vi "Autonomous Independent.vi"   [LabVIEW 2016]
doc: "This VI is called when autonomous begins, and will automatically be terminated when autonomous ends. You can carry out timed or sensor driven robot movement independently without needing to return to the caller."
uses:
  <vilib>/Rock Robotics/WPI/DriverStation/WPI_DriverStationRobotMode2.ctl
  <vilib>/Rock Robotics/WPI/Utilities/WPI_GetSetVariantRefNum.vi
  <vilib>/Rock Robotics/Network Tables/NT Read String.vi
  <vilib>/Rock Robotics/Network Tables/NT Read Number.vi
  Robot Global Data.vi
  <vilib>/Rock Robotics/Network Tables/NT Write Numeric Array.vi
panel:
  # "Be sure to right-click and choose Data Operations>>Make Current Value default if you want to save the array values with the VI"
types:
  T1 = typedef "WPI_JoystickDevRef.ctl" = cluster{"Device":T2}
  T2 = typedef "WPI_JoystickDeviceEnum.ctl" = enum16{"USB 0", "USB 1", "USB 2", "USB 3", "USB 4", "USB 5"}
  T3 = typedef "WPI_DriverStationRobotMode2.ctl" = enum16{"Autonomous Disabled", "Autonomous Enabled", "Teleop Disabled", "Teleop Enabled", "Disconnected", "Finish", "Test Disabled", "Test Enabled", "Emergency Stopped"}
  T4 = typedef "WPI_RobotDriveDevRef.ctl" = cluster{"DevStatus":errorcluster, "Motors[]":T5[], "Square Inputs":bool, "Max Output":dbl}
  T5 = typedef "WPI_MotorControlDeviceRef.ctl" = cluster{"DeviceStatus":errorcluster, "Type":T6, "PWM":cluster{"PWM Channel":T7, "DeadBand":T8}, "CAN":cluster{"Device Number":u8, "SetOutput VI Ref":variant, "GetOutput VI Ref":variant, "Enable VI Ref":variant, "Disable VI Ref":variant, "Data":variant}, "Invert":bool}
  T6 = typedef "WPI_MotorControlType.ctl" = enum16{"PWM", "CAN"}
  T7 = typedef "FPGA_DIOPWMChannel.ctl" = enum8{"PWM 0", "PWM 1", "PWM 2", "PWM 3", "PWM 4", "PWM 5", "PWM 6", "PWM 7", "PWM 8", "PWM 9", "PWM MXP 0", "PWM MXP 1", "PWM MXP 2", "PWM MXP 3", "PWM MXP 4", "PWM MXP 5", "PWM MXP 6", "PWM MXP 7", "PWM MXP 8", "PWM MXP 9", "Invalid"}
  T8 = typedef "WPI_PWMDeadband.ctl" = cluster{"Name":string, "maxPositivePwm":i32, "minPositivePwm":i32, "centerPwm":i32, "maxNegativePwm":i32, "minNegativePwm":i32, "angularRange":u16}
  T9 = typedef "WPI_ServoDeviceRef.ctl" = cluster{"DeviceStatus":errorcluster, "PWM Channel":T7, "DeadBand":T8}
  T10 = typedef "WPI_CANTalonSRX_GlobalStatus.ctl" = cluster{"Applied Throttle":dbl, "Module Enabled":bool, "CAN Error":errorcluster, "Closed Loop Error":dbl, "Forward Limit Switch Closed":bool, "Reverse Limit Switch Closed":bool, "Sensor Position":dbl, "Sensor Velocity":dbl, "Current":dbl, "Sticky Fault - Over Temp":bool, "Sticky Fault - Under Voltage":bool, "Sticky Fault - Forward Limit":bool, "Sticky Fault - Reverse Limit":bool, "Sticky Fault - Forward Soft Limit":bool, "Sticky Fault - Reverse Soft Limit":bool, "Brake is Enabled":bool, "Encoder Position":dbl, "Encoder Velocity":dbl, "Encoder Index Count":dbl, "Encoder A Pin State":bool, "Encoder B Pin State":bool, "Encoder Index Pin State":bool, "Analog In":dbl, "Analog In Velocity":dbl, "Temperature (C)":dbl, "Battery Voltage":dbl, "Control 5 Is Supported":bool, "Current Profile Slot Select":dbl, "Pos Div 8":bool, "Vel Div 4":bool, "Pulse Width Position":i32, "Pulse Width Velocity":i32, "Pulse Width Rise To Rise (us)":i32, "Pulse Width Rise To Fall (us)":i32, "Mot Prof Active Is Under Run":bool, "Mot Prof Active Has Under Run":bool, "Mot Prof Active Is Last":bool, "Mot Prof Active Velocity Only":bool, "Mot Prof Active Is Valid":bool, "Mot Prof Buffer Is Full":bool, "Mot Prof Active Profile Slot Select":i32, "Mot Prof NextID":i32, "Mot Prof Count":i32, "Mot Prof Active Velocity":dbl, "Mot Prof Active Position":dbl, "Mot Prof Output Enable":i32}
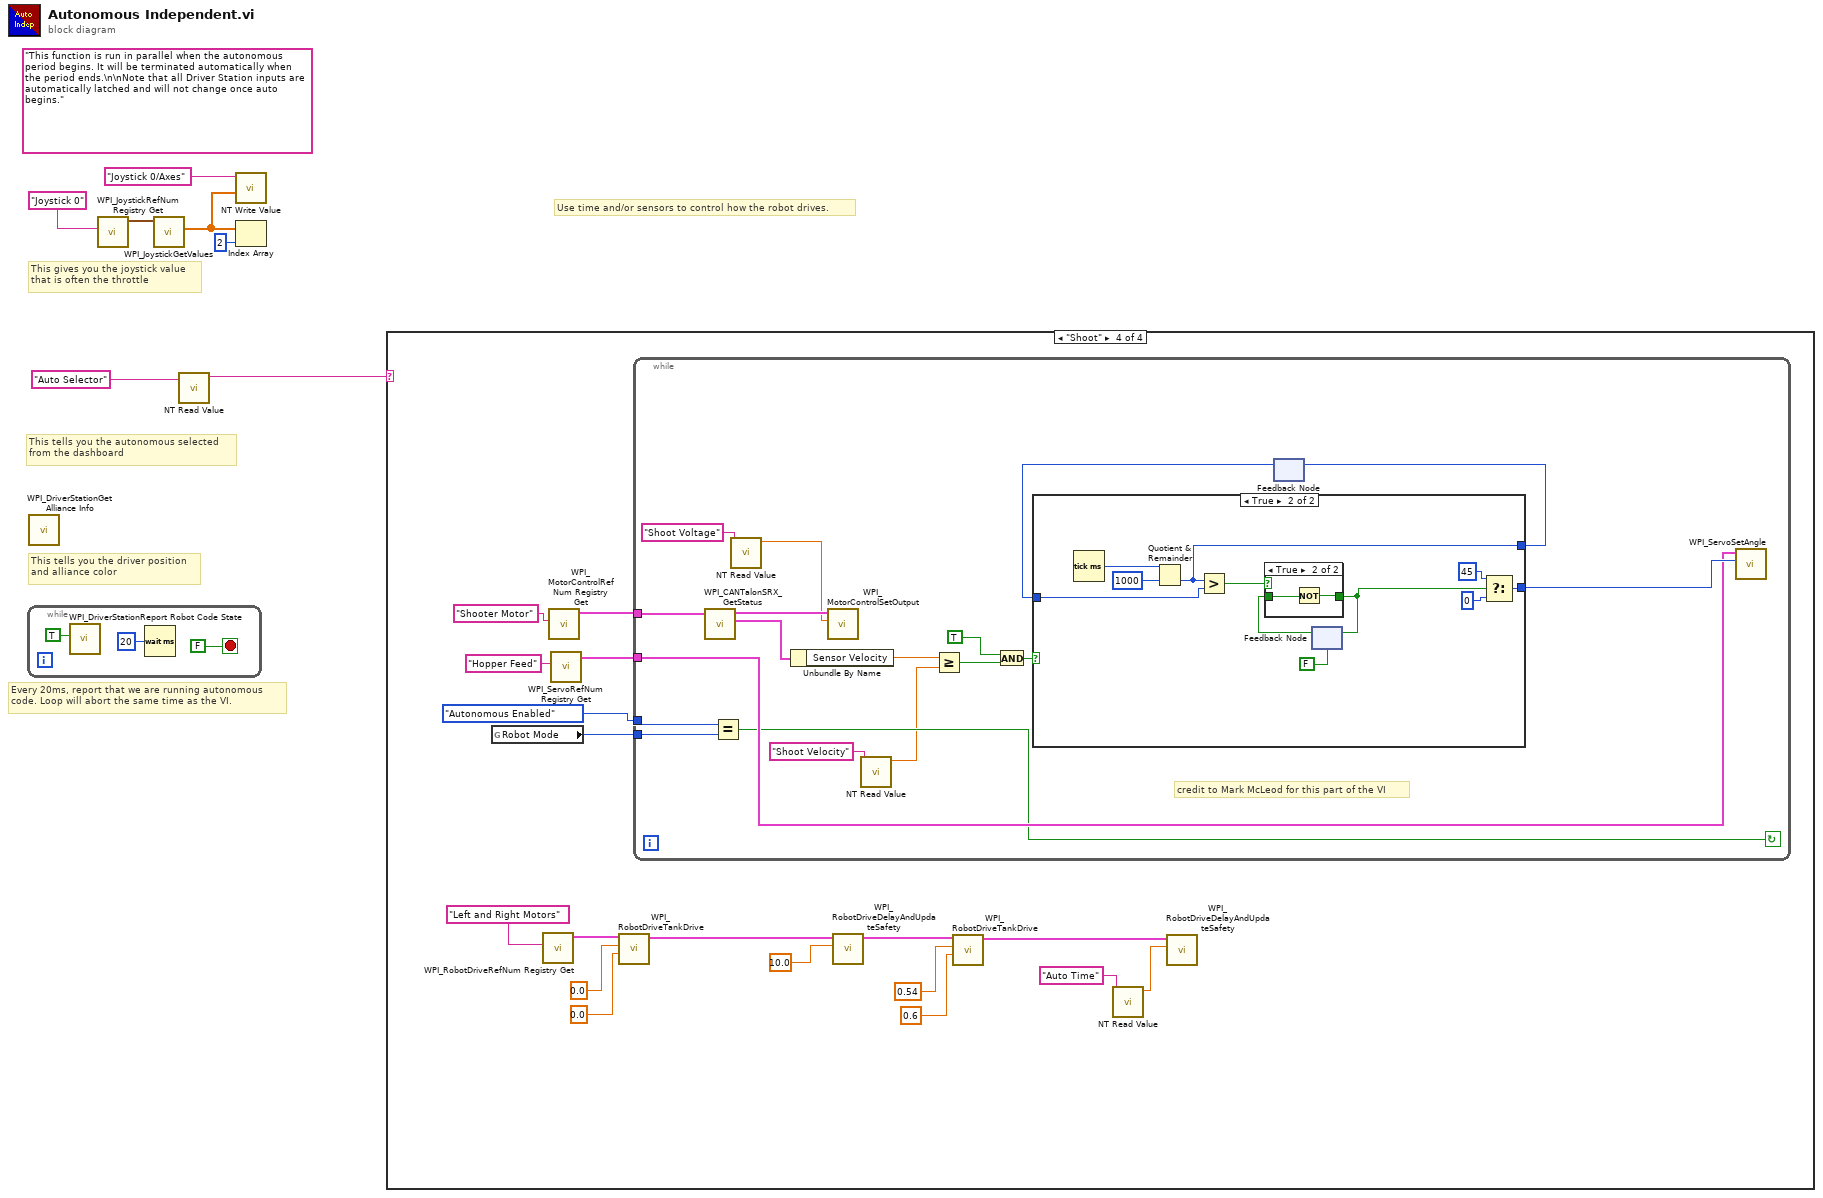
[diagram p0: block diagram]
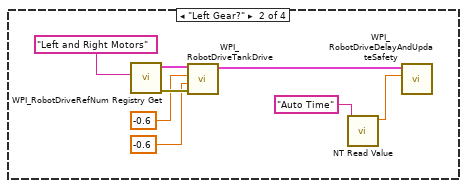
[diagram p3: hidden frame]
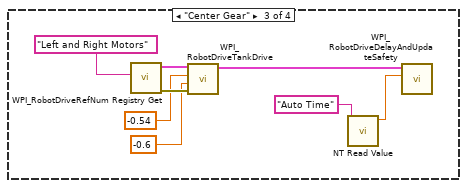
[diagram p4: hidden frame]
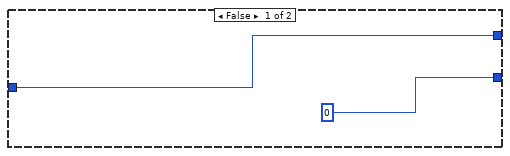
[diagram p5: hidden frame]
diagram:
  (unwired) "This function is run in parallel when the autonomous period begins. It will be terminated automatically when the period ends.\n\nNote that all Driver Station inputs are automatically latched and will not change once auto begins."
  # "This tells you the autonomous selected\nfrom the dashboard"
  # "Every 20ms, report that we are running autonomous\ncode. Loop will abort the same time as the VI."
  # "This gives you the joystick value\nthat is often the throttle"
  # "Use time and/or sensors to control how the robot drives."
  # "This tells you the driver position\nand alliance color"
  n1 = while {
    stop <- FALSE stop-if-true
    n2 = call <vilib>:"WPI_DriverStationReport Robot Code State.vi"("Autonomous"=TRUE) -> ()  [unwired: 10 in, 1 out]
    n3 = Wait (ms)(milliseconds to wait=u32 20) -> ()  [unwired: 1 out]
  }
  n4 = call <vilib>:"WPI_DriverStationGet Alliance Info.vi"() -> ()  [unwired: 12 out]
  n5 = call <vilib>:"WPI_JoystickRefNum Registry Get.vi"("refnum name"="Joystick 0") -> ("JoystickDevRef"=w6:T1)  [unwired: 1 in, 9 out]
  n6 = call <vilib>:"WPI_JoystickGetValues.vi"("JoystickDevRef"=w6) -> ("Axes"=w3:dbl[])  [unwired: 6 in, 4 out]
  n7 = call-poly <vilib>:"NT Read Value.vi"("Name"="Auto Selector") -> ("String"=w1:string)  [unwired: 9 in, 1 out]
  n8 = call-poly <vilib>:"NT Write Value.vi"("Numeric Array"=w3, "Name"="Joystick 0/Axes") -> ()  [unwired: 9 in, 1 out]
  n9 = Index Array(array=w3, index=2) -> ()  [unwired: 1 out]
  n10 = case shown="\"Shoot\"" w1 {
    frame Default {
    }
    frame "Left Gear?" {
      n11 = call <vilib>:"WPI_RobotDriveRefNum Registry Get.vi"("refnum name"="Left and Right Motors") -> ("error out"=w17:errorcluster, "RobotDriveDevRef"=w16:T4)  [unwired: 1 in, 8 out]
      n12 = call <vilib>:"WPI_RobotDriveTankDrive.vi"("error in (no error)"=w17, "Right axis value"=-0.6, "Left axis value"=-0.6, "RobotDriveDevRef"=w16) -> ("RobotDriveDevRef"=w13:T4)  [unwired: 5 in, 2 out]
      n13 = call-poly <vilib>:"NT Read Value.vi"("Name"="Auto Time") -> ("Numeric"=w12:dbl)  [unwired: 9 in, 1 out]
      n14 = call <vilib>:"WPI_RobotDriveDelayAndUpdateSafety.vi"("Delay (s)"=w12, "RobotDriveDevRef"=w13) -> ()  [unwired: 8 in, 2 out]
    }
    frame "Center Gear" {
      n15 = call <vilib>:"WPI_RobotDriveRefNum Registry Get.vi"("refnum name"="Left and Right Motors") -> ("error out"=w25:errorcluster, "RobotDriveDevRef"=w24:T4)  [unwired: 1 in, 8 out]
      n16 = call <vilib>:"WPI_RobotDriveTankDrive.vi"("error in (no error)"=w25, "Right axis value"=-0.6, "Left axis value"=-0.54, "RobotDriveDevRef"=w24) -> ("RobotDriveDevRef"=w21:T4)  [unwired: 5 in, 2 out]
      n17 = call-poly <vilib>:"NT Read Value.vi"("Name"="Auto Time") -> ("Numeric"=w20:dbl)  [unwired: 9 in, 1 out]
      n18 = call <vilib>:"WPI_RobotDriveDelayAndUpdateSafety.vi"("Delay (s)"=w20, "RobotDriveDevRef"=w21) -> ()  [unwired: 8 in, 2 out]
    }
    frame "Shoot" {
      n19 = global read "Robot Global Data.vi" "Robot Mode"() -> (w40:T3)
      n20 = call <vilib>:"WPI_RobotDriveRefNum Registry Get.vi"("refnum name"="Left and Right Motors") -> ("RobotDriveDevRef"=w28:T4)  [unwired: 1 in, 9 out]
      n21 = call <vilib>:"WPI_MotorControlRefNum Registry Get.vi"("refnum name"="Shooter Motor") -> ("MotorControlDevRef"=w43:T5)  [unwired: 9 in, 1 out]
      n22 = call <vilib>:"WPI_ServoRefNum Registry Get.vi"("refnum name"="Hopper Feed") -> ("ServoDeviceRef"=w41:T9)  [unwired: 9 in, 1 out]
      n23 = call <vilib>:"WPI_RobotDriveTankDrive.vi"("Right axis value"=0.0, "Left axis value"=0.0, "RobotDriveDevRef"=w28) -> ("RobotDriveDevRef"=w30:T4)  [unwired: 6 in, 2 out]
      n24 = while {
        tunnel: w43 -> [w59]
        tunnel: w41 -> [w52]
        tunnel: WPI_DriverStationRobotMode2."Autonomous Enabled" ("Robot Mode") -> [w51]
        tunnel: w40 -> [w50]
        stop <- w49 continue-if-true
        # "credit to Mark McLeod for this part of the VI"
        n25 = call <vilib>:"WPI_CANTalonSRX_GetStatus.vi"("CAN Talon SRX Ref"=w59) -> ("Talon SRX Status"=w61:T10, "CAN Talon SRX Ref"=w62:T5)  [unwired: 8 in, 1 out]
        n26 = Equal?(x=w51, y=w50) -> (x = y?=w49:bool)
        n27 = call-poly <vilib>:"NT Read Value.vi"("Name"="Shoot Voltage") -> ("Numeric"=w45:dbl)  [unwired: 9 in, 1 out]
        n28 = Unbundle By Name(w61) -> ("Sensor Velocity"=w60:dbl)
        n29 = call <vilib>:"WPI_MotorControlSetOutput.vi"("Output"=w45, "MotorControlDevRef"=w62) -> ()  [unwired: 7 in, 3 out]
        n30 = call-poly <vilib>:"NT Read Value.vi"("Name"="Shoot Velocity") -> ("Numeric"=w48:dbl)  [unwired: 9 in, 1 out]
        n31 = Greater Or Equal?(x=w60, y=w48) -> (x >= y?=w53:bool)
        n32 = And(x=TRUE, y=w53) -> (x .and. y?=w56:bool)
        n33 = feedback #1() -> (w57:u32)  [unwired: 1 in]
        n34 = case shown="True" w56 {
          tunnel: [0 ("Angle") w75] -> w55
          tunnel: w57 -> [w63 w66]
          tunnel: [w63 w65] -> w58
          frame False {
          }
          frame True {
            n35 = Tick Count (ms)() -> (millisecond timer value=w72:u32)
            n36 = Quotient & Remainder(x=w72, y=u32 1000) -> (floor(x/y)=w65:u32)  [unwired: 1 out]
            n37 = Greater?(x=w65, y=w66) -> (0:w67:bool)
            n38 = feedback #2(FALSE) -> (w69:bool)
            n39 = case shown="True" w67 {
              tunnel: w69 -> [w76 w78]
              tunnel: [w76 w77] -> w70
              frame False {
              }
              frame True {
                n40 = Not(x=w78) -> (.not. x?=w77:bool)
              }
            }
            n41 = feedback-in #2(w70) -> ()
            n42 = Select(t=45 ("Angle"), s=w70, f=0 ("Angle")) -> (s? t:f=w75:i32)
          }
        }
        n43 = feedback-in #1(w58) -> ()
        n44 = call <vilib>:"WPI_ServoSetAngle.vi"("Angle"=w55, "ServoDeviceRef"=w52) -> ()  [unwired: 8 in, 2 out]
      }
      n45 = call <vilib>:"WPI_RobotDriveDelayAndUpdateSafety.vi"("Delay (s)"=10.0, "RobotDriveDevRef"=w30) -> ("RobotDriveDevRef 2"=w29:T4)  [unwired: 8 in, 1 out]
      n46 = call <vilib>:"WPI_RobotDriveTankDrive.vi"("Right axis value"=0.6, "Left axis value"=0.54, "RobotDriveDevRef"=w29) -> ("RobotDriveDevRef"=w36:T4)  [unwired: 6 in, 2 out]
      n47 = call-poly <vilib>:"NT Read Value.vi"("Name"="Auto Time") -> ("Numeric"=w35:dbl)  [unwired: 9 in, 1 out]
      n48 = call <vilib>:"WPI_RobotDriveDelayAndUpdateSafety.vi"("Delay (s)"=w35, "RobotDriveDevRef"=w36) -> ()  [unwired: 8 in, 2 out]
    }
  }
